vi "BuildResetHardwareString.vi"(10 "String":string[](array[string])=["Flow Instrument Initial Failed！", "Hengyuan Pressure Initial Failed！", "Connection PLC Failed！"], 11 "Error":bool[](array[boolean])) -> (3 "DataOut":string)   [LabVIEW 2017]
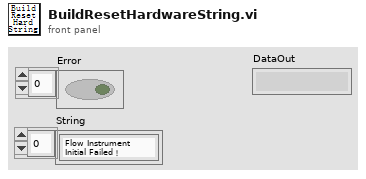
[diagram p1: front panel]
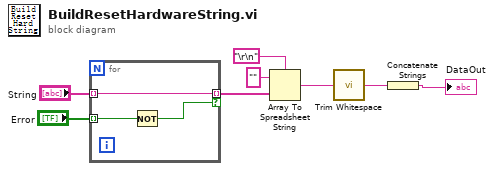
[diagram p0: block diagram]
diagram:
  n1 = for {
    tunnel: "String" -> [w11] mode=indexing
    tunnel: [w11] -> w6 mode=indexing if=w9
    tunnel: "Error" -> [w10] mode=indexing
    n2 = Not(x=w10) -> (.not. x?=w9:bool)
  }
  n3 = Array To Spreadsheet String(delimiter (Tab)="\r\n", array=w6, 3:"" ("format string")) -> (spreadsheet string=w4:string)
  n4 = call <vilib>:"Trim Whitespace.vi"("string"=w4) -> ("trimmed string"=w3:string)  [unwired: 1 in]
  n5 = Concatenate Strings(w3) -> (→"DataOut":string)
